vi "AssertNotEqual_Tests.vi"(11 "error in (no error)":errorcluster) -> (15 "error out":errorcluster)   [LabVIEW 2016, in "DronaTest.lvlib"]
uses:
  DronaTest.lvlib
  APIs/Assert/AssertControlValue/NotEqual.vi
  <vilib>/addons/_JKI Toolkits/Caraya/classes/Assert/Assert Error.vi
  <vilib>/addons/_JKI Toolkits/Caraya/classes/Assert/Assert Not Equal Value_Variant.vi
  <vilib>/addons/_JKI Toolkits/Caraya/classes/Test/Test.lvclass
  Drona.lvlib
  <vilib>/addons/_JKI Toolkits/Caraya/classes/Assert/Assert.lvclass
  APIs/Assert/AssertControlValue/AssertControlValue.lvlib
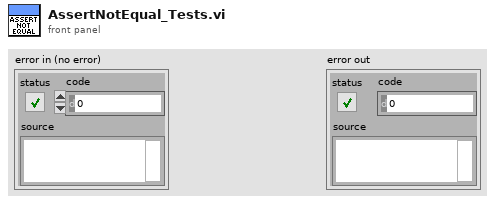
[diagram p1: front panel]
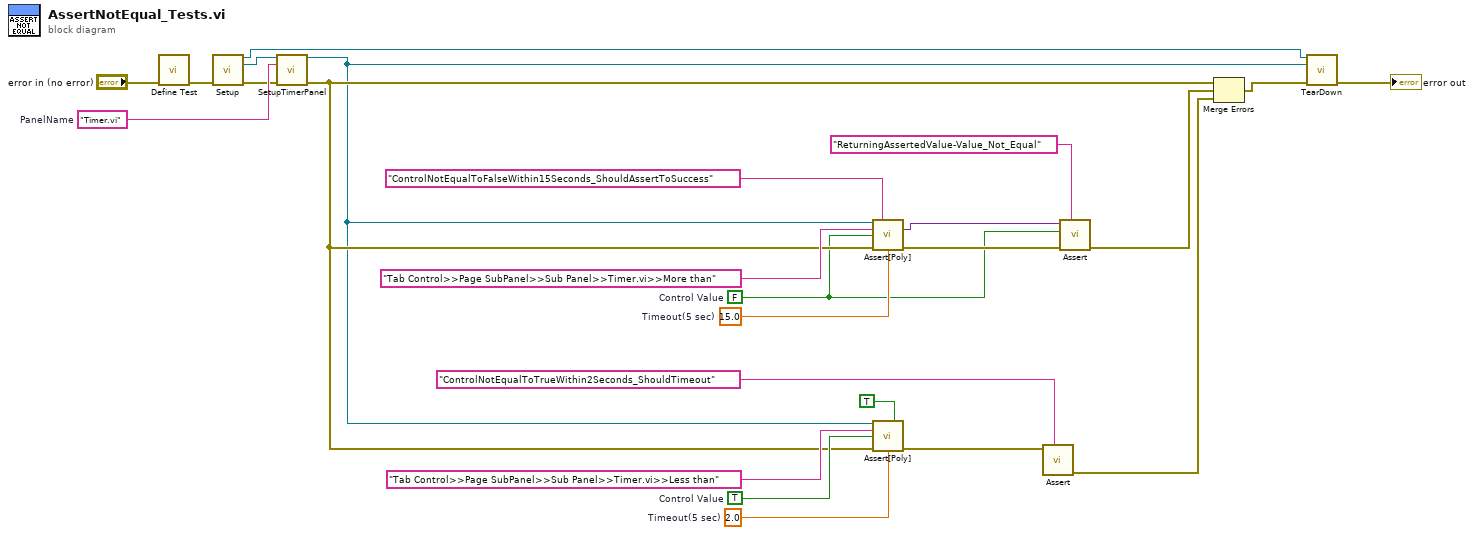
[diagram p0: block diagram]
diagram:
  w14 = "Timer.vi"  # PanelName
  w15 = TRUE  # Control Value
  w20 = 2.0  # Timeout(5 sec)
  w19 = 15.0  # Timeout(5 sec)
  w1 = FALSE  # Control Value
  n1 = call <vilib>:"Define Test.vi"("error in (no error)"="error in (no error)") -> ("error out"=w13:errorcluster)  [unwired: 10 in]
  n2 = call "Setup.vi"("error in (no error)"=w13) -> ("Application Ref"=w10:refnum<vi>, "VI out"=w11:refnum<vi>, "error out"=w12:errorcluster)  [unwired: 12 in]
  n3 = call "SetupTimerPanel.vi"("VI in"=w11, "Panel Name"=w14, "error in (no error)"=w12) -> ("VI out"=w6:refnum<vi>, "error out"=w9:errorcluster)  [unwired: 11 in]
  n4 = call-poly "Assert[Poly].vi"("VI Reference In"=w6, "Test Label"="ControlNotEqualToFalseWithin15Seconds_ShouldAssertToSuccess" ("string"), "Control Path"="Tab Control>>Page SubPanel>>Sub Panel>>Timer.vi>>More than", "Control Value"=w1, "Error In"=w9, "Timeout(5 sec)"=w19) -> ("Asserted Value"=w2:variant, "Error Out"=w5:errorcluster)  [unwired: 7 in, 1 out]
  n5 = call-poly "Assert[Poly].vi"("VI Reference In"=w6, "Assert Only? (F)"=TRUE, "Control Path"="Tab Control>>Page SubPanel>>Sub Panel>>Timer.vi>>Less than", "Control Value"=w15, "Error In"=w9, "Timeout(5 sec)"=w20) -> ("Error Out"=w22:errorcluster)  [unwired: 7 in, 2 out]
  n6 = call-poly <vilib>:"Assert.vi"("Label"="ControlNotEqualToTrueWithin2Seconds_ShouldTimeout" ("string"), "Error?"=w22) -> ("error out"=w16:errorcluster)  [unwired: 9 in]
  n7 = call-poly <vilib>:"Assert.vi"("Label"="ReturningAssertedValue-Value_Not_Equal", "error in (no error)"=w5, "Y"=w1, "X"=w2) -> ("error out"=w4:errorcluster)  [unwired: 7 in]
  n8 = Merge Errors(w9, w4, w16) -> (w8:errorcluster)
  n9 = call "TearDown.vi"("Application Ref"=w10, "VI in"=w6, "error in (no error)"=w8) -> ("error out"=→"error out":errorcluster)  [unwired: 12 in]
